vi "visibleOrIR.vi"(7 "Monochromator":T2={"Type"=enum."PTI", "Wavelength (nm)"=600.0, "Grating, gr/mm"=enum."1200", "Grating mode"=enum."Unknown", "Spectrum mode"={"Spectrum mode?"=FALSE, "Start wavelength (nm)"=0.0, "End wavelength (nm)"=0.0, "Wavelength step (nm)"=0.0, "Wavelength array"=[], "array index"=0}, "PTI"={"Delay before read (ms)"=50, "Mono 1"={"Timeout (ms)"=1000, "Resource Name"="COM1", "Baud Rate"=9600, "Data Bits"=8, "Parity"=0, "Stop Bits"=10, "Flow Control"=0}, "Mono 2"={"Timeout (ms)"=1000, "Resource Name"="COM1", "Baud Rate"=9600, "Data Bits"=8, "Parity"=0, "Stop Bits"=10, "Flow Control"=0}, "Two PTI Monochromators?"=FALSE}, "Oriel (custom)"={"reference"=refnum}, "Force wavelength confirmation (PTI)?"=FALSE} {"PTI"."Mono 2"."Flow Control" items=["1.0"=10, "1.5"=15, "2.0"=20]; "PTI"."Mono 2"."Stop Bits" items=["None", "Odd", "Even", "Mark", "Space"]; "PTI"."Mono 2"."Parity" items=["None", "Odd", "Even", "Mark", "Space"]; "PTI"."Mono 1"."Flow Control" items=["1.0"=10, "1.5"=15, "2.0"=20]; "PTI"."Mono 1"."Stop Bits" items=["None", "Odd", "Even", "Mark", "Space"]; "PTI"."Mono 1"."Parity" items=["None", "Odd", "Even", "Mark", "Space"]}, 11 "Wavelength (nm)":dbl) -> (1 "Grating, gr/mm":T1, 2 "IR/visible":T4=enum."IR", 3 "Displayed mono wavelength (nm)":dbl)   [LabVIEW 2017, in "Monochromator.lvlib"]
uses:
  Monochromator.lvlib
  Controls/Grating.ctl
  Controls/Params.ctl
  Controls/Type.ctl
  Controls/GratingValues.ctl
  PTI/Controls/Params.ctl
  Controls/VISA parameters.ctl
  Custom Oriel drivers/Controls/Params.ctl
  C:/Project Work/icl-optical-software-rewrite/Optical Software Code Simplified/Modules/Monochromator/Cornerstone.dll
  Cornerstone.dll
  Serial comms/Serial comms.lvlib
  PTI/PTI.lvlib
  Custom Oriel drivers/Oriel (custom drivers).lvlib
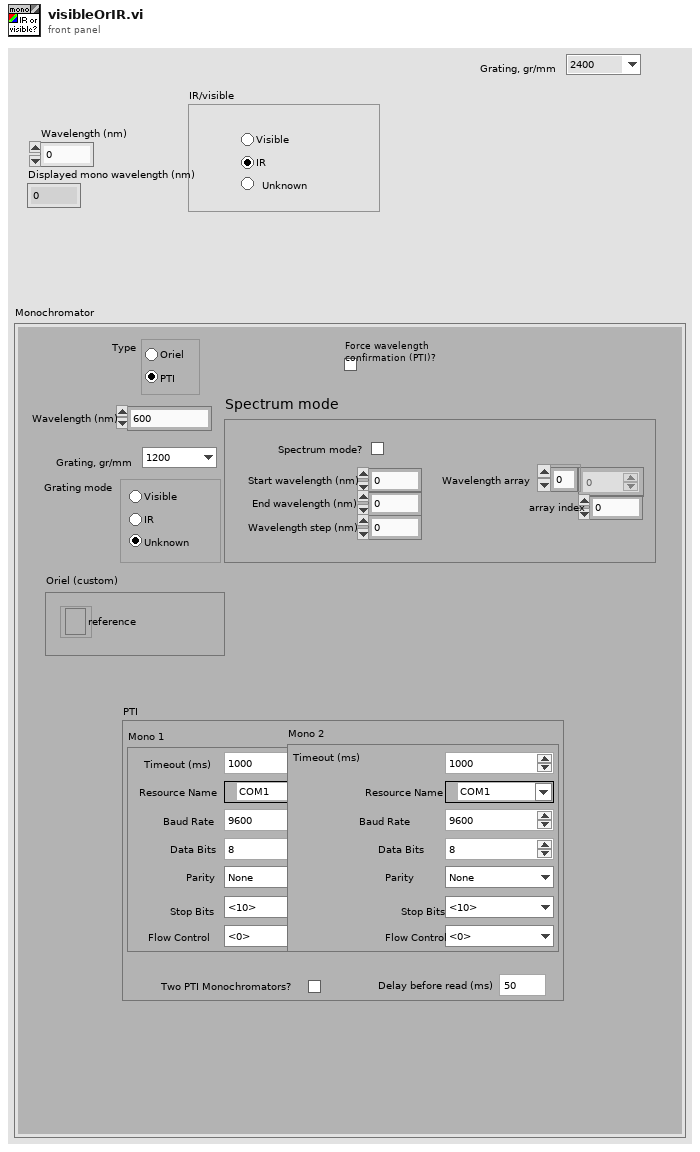
[diagram p1: front panel]
types:
  T1 = typedef "Monochromator.lvlib/GratingValues.ctl" = enum16{"2400", "1800", "1200", "600", "300", "150"}
  T2 = typedef "Monochromator.lvlib/Params.ctl" = cluster{"Type":T3, "Wavelength (nm)":dbl, "Grating, gr/mm":T1, "Grating mode":T4, "Spectrum mode":cluster{"Spectrum mode?":bool, "Start wavelength (nm)":dbl, "End wavelength (nm)":dbl, "Wavelength step (nm)":dbl, "Wavelength array":dbl[], "array index":u32}, "PTI":T5, "Oriel (custom)":T7, "Force wavelength confirmation (PTI)?":bool}
  T3 = typedef "Monochromator.lvlib/Type.ctl" = enum32{"Oriel", "PTI"}
  T4 = typedef "Monochromator.lvlib/Grating.ctl" = enum32{"Unknown", "Visible", "IR"}
  T5 = typedef "Monochromator.lvlib/PTI.lvlib/Params.ctl" = cluster{"Delay before read (ms)":u32, "Mono 1":T6, "Mono 2":T6, "Two PTI Monochromators?":bool}
  T6 = typedef "Serial comms.lvlib/VISA parameters.ctl" = cluster{"Timeout (ms)":u32, "Resource Name":refnum<visa-resource-name>, "Baud Rate":u32, "Data Bits":u16, "Parity":u16, "Stop Bits":u16, "Flow Control":u16}
  T7 = typedef "Monochromator.lvlib/Oriel (custom drivers).lvlib/Params.ctl" = cluster{"reference":refnum<k24>}
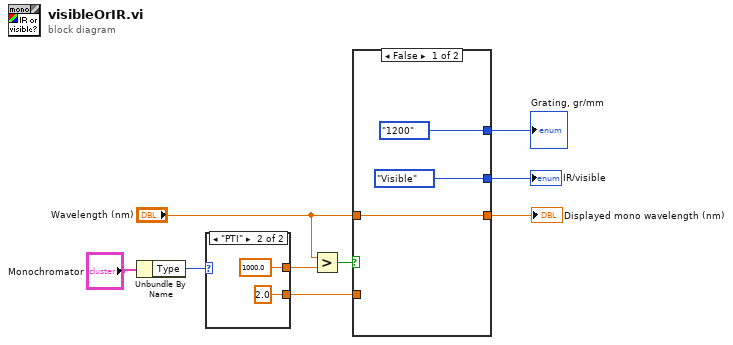
[diagram p0: block diagram]
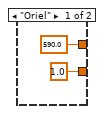
[diagram p2: hidden frame]
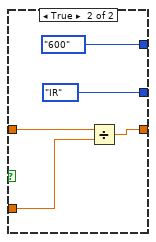
[diagram p3: hidden frame]
diagram:
  n1 = Unbundle By Name("Monochromator") -> ("Type"=w6:T3)
  n2 = case shown="\"PTI\"" w6 {
    tunnel: [590.0 ("y") 1000.0 ("y")] -> w5
    tunnel: [1.0 ("y") 2.0 ("y")] -> w3
    frame "Oriel" {
    }
    frame "PTI" {
    }
  }
  n3 = Greater?(x="Wavelength (nm)", y=w5) -> (0:w4:bool)
  n4 = case shown="False" w4 {
    tunnel: [Grating."Visible" ("Grating") Grating."IR" ("Grating")] -> w9
    tunnel: "Wavelength (nm)" -> [w15 w19]
    tunnel: [w15 w20] -> w7
    tunnel: w3 -> [_ w18]
    tunnel: [GratingValues."1200" ("Grating, gr/mm") GratingValues."600" ("Grating, gr/mm")] -> w1
    frame False {
    }
    frame True {
      n5 = Divide(x=w19, y=w18) -> (x/y=w20:dbl)
    }
  }
  "IR/visible" <- w9
  "Displayed mono wavelength (nm)" <- w7
  "Grating, gr/mm" <- w1
